vi "Elapsed Time.vi"() -> (0 "Rate (s-1)":dbl format="%#_3g")   [LabVIEW 2023]
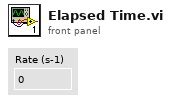
[diagram p1: front panel]
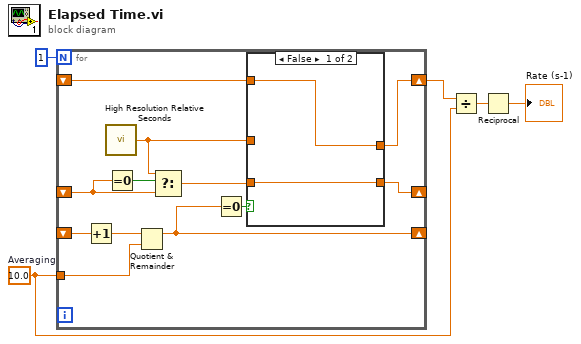
[diagram p0: block diagram]
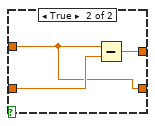
[diagram p2: hidden frame]
diagram:
  w1 = 10.0  # Averaging
  n1 = for {
    N: 1 -> [_]
    shift-right: [w12] -> _
    shift-left: _ -> [w16]
    shift-right: [w6] -> _
    shift-left: _ -> [w15]
    tunnel: w1 -> [w14]
    shift-right: [w10] -> w3
    shift-left: _ -> [w9]
    n2 = Increment(x=w15) -> (x+1=w7:dbl)
    n3 = call <vilib>:"High Resolution Relative Seconds.vi"() -> ("relative seconds"=w11:dbl)
    n4 = Equal To 0?(x=w16) -> (x = 0?=w17:bool)
    n5 = Quotient & Remainder(x=w7, y=w14) -> (x-y*floor(x/y)=w6:dbl)  [unwired: 1 out]
    n6 = Select(t=w11, s=w17, f=w16) -> (s? t:f=w13:dbl)
    n7 = Equal To 0?(x=w6) -> (x = 0?=w8:bool)
    n8 = case shown="False" w8 {
      tunnel: w13 -> [w19 w21]
      tunnel: [w19 w20] -> w12
      tunnel: w11 -> [_ w20]
      tunnel: [w18 w22] -> w10
      tunnel: w9 -> [w18 _]
      frame False {
      }
      frame True {
        n9 = Subtract(x=w20, y=w21) -> (x-y=w22:dbl)
      }
    }
  }
  n10 = Divide(x=w3, y=w1) -> (x/y=w2:dbl)
  n11 = Reciprocal(x=w2) -> (1/x=→"Rate (s-1)":dbl)
